vi "mod_Sample & Hold BitStream.vi"(0 "input bit stream":u8[](array[numeric]), 5 "samples per bit":i32=1, 7 "Optimize for":enum16{"Speed", "Memory", "Speed & Memory"}(ring)) -> (4 "upsampled bit stream":u8[](array[numeric]))   [LabVIEW 2020, in "niAMT.lvlib"]
uses:
  <vilib>/addons/Modulation/niAMT.lvlib
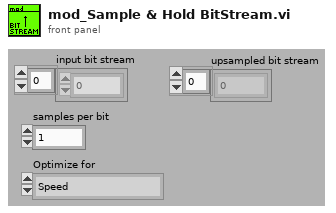
[diagram p1: front panel]
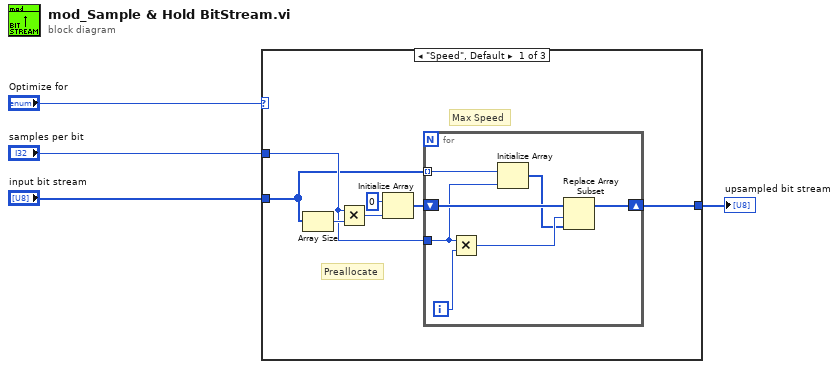
[diagram p0: block diagram]
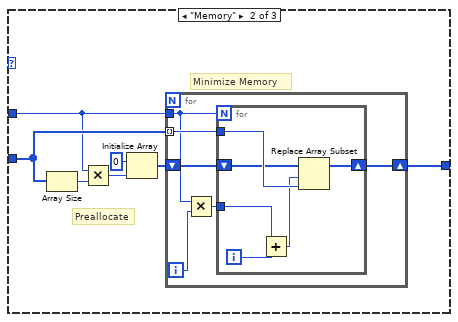
[diagram p2: hidden frame]
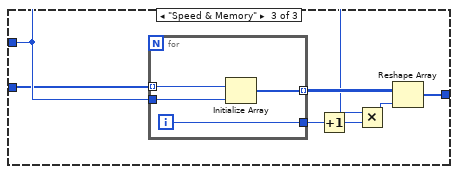
[diagram p3: hidden frame]
diagram:
  n1 = case shown="\"Speed\", Default" "Optimize for" {
    tunnel: "input bit stream" -> [w5 w21 w39]
    tunnel: [w11 w25 w38] -> w3
    tunnel: "samples per bit" -> [w6 w20 w40]
    frame "Speed", Default {
      # "Preallocate"
      # "Max Speed"
      n2 = Array Size(array=w5) -> (size(s)=w10:i32)
      n3 = Multiply(x=w6, y=w10) -> (x*y=w8:i32)
      n4 = Initialize Array(u8 0 ("element"), w8) -> (w7:u8[])
      n5 = for {
        tunnel: w5 -> [w14] mode=indexing
        shift-right: [w17] -> w11
        shift-left: w7 -> [w18]
        tunnel: w6 -> [w13]
        i -> [w16]
        n6 = Multiply(x=w13, y=w16) -> (x*y=w15:i32)
        n7 = Initialize Array(w14, w13) -> (w12:u8[])
        n8 = Replace Array Subset(array=w18, new element=w12, index=w15) -> (w17:u8[])
      }
    }
    frame "Memory" {
      # "Preallocate"
      # "Minimize Memory"
      n9 = Array Size(array=w21) -> (size(s)=w24:i32)
      n10 = Multiply(x=w20, y=w24) -> (x*y=w22:i32)
      n11 = Initialize Array(u8 0 ("element"), w22) -> (w19:u8[])
      n12 = for {
        tunnel: w20 -> [w26]
        tunnel: w21 -> [w30] mode=indexing
        shift-right: [w29] -> w25
        shift-left: w19 -> [w31]
        i -> [w28]
        n13 = Multiply(x=w26, y=w28) -> (x*y=w27:i32)
        n14 = for {
          N: w26 -> [_]
          shift-right: [w35] -> w29
          shift-left: w31 -> [w36]
          tunnel: w30 -> [w37]
          tunnel: w27 -> [w33]
          i -> [w34]
          n15 = Add(x=w33, y=w34) -> (x+y=w32:i32)
          n16 = Replace Array Subset(array=w36, new element=w37, index=w32) -> (w35:u8[])
        }
      }
    }
    frame "Speed & Memory" {
      n17 = for {
        tunnel: w39 -> [w48] mode=indexing
        tunnel: w40 -> [w47]
        tunnel: [w46] -> w44 mode=indexing
        tunnel: [w45] -> w43
        i -> [w45]
        n18 = Initialize Array(w48, w47) -> (w46:u8[])
      }
      n19 = Increment(x=w43) -> (x+1=w41:i32)
      n20 = Multiply(x=w40, y=w41) -> (x*y=w42:i32)
      n21 = Reshape Array(w44, w42) -> (w38:u8[])
    }
  }
  "upsampled bit stream" <- w3
